vi "SectionA04_Week6_Stus.vi"() -> ()   [LabVIEW 2013]
panel:
  in  "?":bool
  in  "multiply":bool
  in  "divide":bool
  in  "subtract":bool
  in  "add":bool
  out "answer":dbl
  in  "Y":dbl
  in  "X":dbl
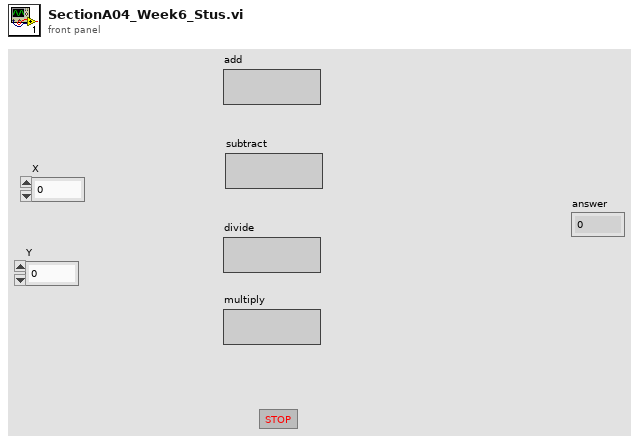
[diagram p1: front panel]
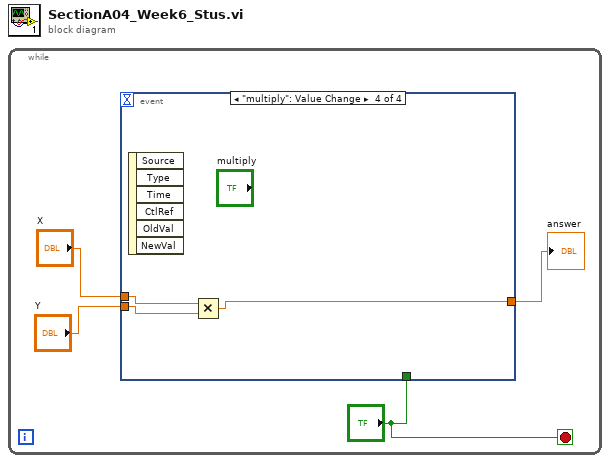
[diagram p0: block diagram]
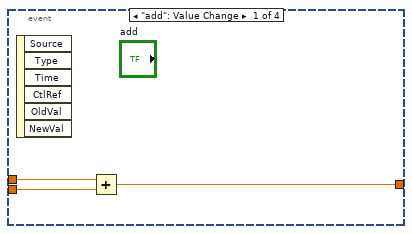
[diagram p2: hidden frame]
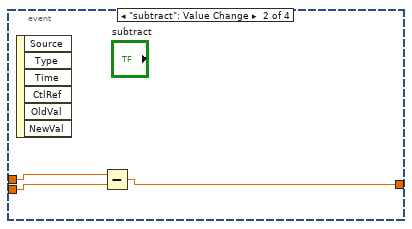
[diagram p3: hidden frame]
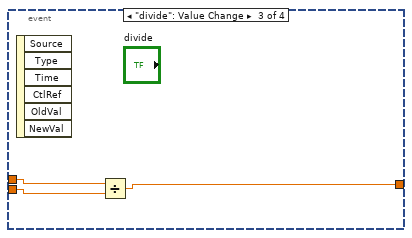
[diagram p4: hidden frame]
diagram:
  n1 = while {
    stop <- "?" stop-if-true
    n2 = event shown="[3] \"multiply\": Value Change" {
      selector: _ -> [_ _ _ _]
      dyn-events: _ -> [_ _ _ _]
      timeout: _ -> [_ _ _ _]
      tunnel: "X" -> [w7 w10 w13 w16]
      tunnel: "Y" -> [w6 w9 w12 w15]
      tunnel: [w5 w8 w11 w14] -> w2
      tunnel: "?" -> [_ _ _ _]
      event "add": Value Change {
        n3 = event-data() -> ()  [unwired: 1 in, 6 out]
        n4 = Add(x=w7, y=w6) -> (x+y=w5:dbl)
      }
      event "subtract": Value Change {
        n5 = event-data() -> ()  [unwired: 1 in, 6 out]
        n6 = Subtract(x=w10, y=w9) -> (x-y=w8:dbl)
      }
      event "divide": Value Change {
        n7 = event-data() -> ()  [unwired: 1 in, 6 out]
        n8 = Divide(x=w13, y=w12) -> (x/y=w11:dbl)
      }
      event "multiply": Value Change {
        n9 = event-data() -> ()  [unwired: 1 in, 6 out]
        n10 = Multiply(x=w16, y=w15) -> (x*y=w14:dbl)
      }
    }
    "answer" <- w2
  }
